vi "rad7_subvi.vi"(8 "error in (no error)":errorcluster, 11 "VISA resource name":refnum<visa-resource-name>) -> (0 "error out":errorcluster, 1 "Rad7 data":dbl, 2 "Rad7 data":string, 3 "VISA resource name out":refnum<visa-resource-name>)   [LabVIEW 2012]
panel:
  out "Numeric 3":i32
  out "read buffer":string
  out "millisecond timer value":u32
  out "Numeric 2":i32
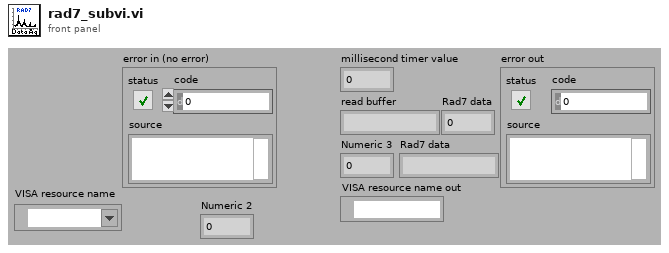
[diagram p1: front panel]
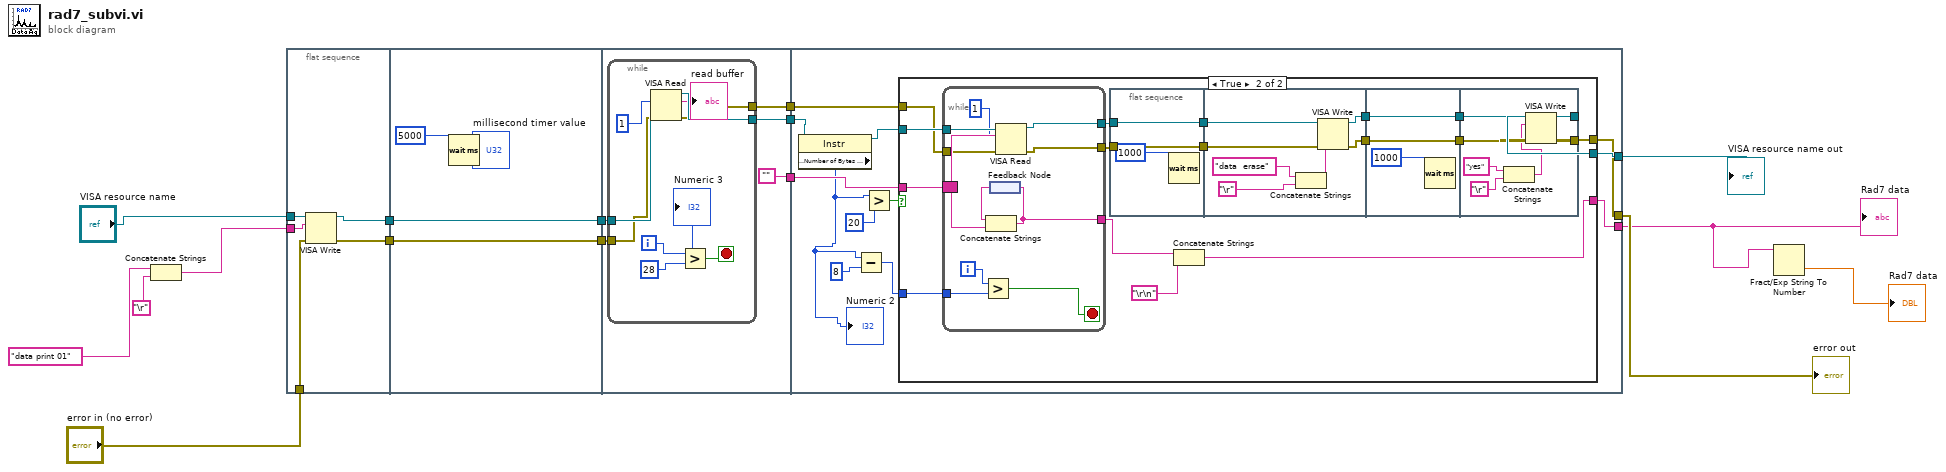
[diagram p0: block diagram]
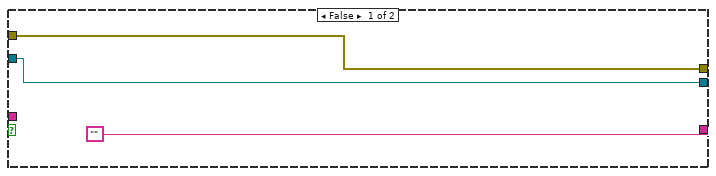
[diagram p2: hidden frame]
diagram:
  n1 = Concatenate Strings("data print 01" ("Command"), "\r") -> (w7:string)
  n2 = flat-sequence {
    tunnel: w7 -> [w21]
    tunnel: [w20] -> w16
    tunnel: [w19] -> w15
    tunnel: "error in (no error)" -> [w18]
    tunnel: "VISA resource name" -> [w17]
    tunnel: w16 -> [w25]
    tunnel: [w25] -> w14
    tunnel: w15 -> [w24]
    tunnel: [w24] -> w13
    tunnel: [w30] -> w12
    tunnel: [""] -> w11
    tunnel: [w28] -> w10
    tunnel: w14 -> [w27]
    tunnel: w13 -> [w26]
    tunnel: [w51] -> w5
    tunnel: w12 -> [w49]
    tunnel: w11 -> [w50]
    tunnel: [w43] -> w2
    tunnel: w10 -> [w45]
    tunnel: [w44] -> w6
    frame #0 {
      n3 = VISA Write(VISA resource name=w17, write buffer=w21, error in (no error)=w18) -> (VISA resource name out=w20:refnum<visa-resource-name>, error out=w19:errorcluster)  [unwired: 1 out]
    }
    frame #1 {
      n4 = Wait (ms)(milliseconds to wait=5000) -> (millisecond timer value=→"millisecond timer value":u32)
    }
    frame #2 {
      n5 = while {
        tunnel: w27 -> [w38]
        tunnel: [w34] -> w30
        tunnel: w26 -> [w33]
        tunnel: [w32] -> w28
        i -> [w37]
        stop <- w35 stop-if-true
        n6 = VISA Read(VISA resource name=w38, byte count=1, error in (no error)=w33) -> (VISA resource name out=w34:refnum<visa-resource-name>, read buffer=→"read buffer":string, error out=w32:errorcluster)  [unwired: 1 out]
        n7 = Greater?(x=w37, y=28) -> (0:w35:bool)
        "Numeric 3" <- w37
      }
    }
    frame #3 {
      n8 = property class="Instr"(reference=w49) -> (reference out=w48:refnum<visa-resource-name>, "Serial Settings:Number of Bytes at Serial Port"=w40:u32)  [unwired: 1 in, 1 out]
      "Numeric 2" <- w40
      n9 = Subtract(x=w40, y=8) -> (x-y=w41:u32)
      n10 = Greater?(x=w40, y=20) -> (0:w47:bool)
      n11 = case shown="True" w47 {
        tunnel: [w54 w65] -> w51
        tunnel: w50 -> [_ w71]
        tunnel: ["" w57] -> w43
        tunnel: w48 -> [w54 w70]
        tunnel: w41 -> [_ w69]
        tunnel: w45 -> [w53 w64]
        tunnel: [w53 w62] -> w44
        frame False {
        }
        frame True {
          n12 = while {
            tunnel: w70 -> [w98]
            border: w71 -> [_]
            tunnel: [w99] -> w67
            tunnel: w69 -> [w96]
            tunnel: [w94] -> w66
            tunnel: w64 -> [w93]
            tunnel: [w92] -> w63
            i -> [w100]
            stop <- w95 stop-if-true
            n13 = Greater?(x=w100, y=w96) -> (0:w95:bool)
            n14 = feedback #1() -> (w101:string)
            n15 = VISA Read(VISA resource name=w98, byte count=1, error in (no error)=w93) -> (VISA resource name out=w94:refnum<visa-resource-name>, read buffer=w102:string, error out=w92:errorcluster)  [unwired: 1 out]
            n16 = Concatenate Strings(w101, w102) -> (w99:string)
            n17 = feedback-in #1(w99) -> ()
          }
          n18 = flat-sequence {
            tunnel: w63 -> [w73]
            tunnel: w66 -> [w74]
            tunnel: [w74] -> w56
            tunnel: [w73] -> w55
            tunnel: [w78] -> w61
            tunnel: [w75] -> w59
            tunnel: w56 -> [w77]
            tunnel: w55 -> [w76]
            tunnel: w61 -> [w84]
            tunnel: [w84] -> w60
            tunnel: w59 -> [w83]
            tunnel: [w83] -> w58
            tunnel: w60 -> [w88]
            tunnel: [w87] -> w65
            tunnel: w58 -> [w86]
            tunnel: [w85] -> w62
            frame #0 {
              n19 = Wait (ms)(milliseconds to wait=1000) -> ()  [unwired: 1 out]
            }
            frame #1 {
              n20 = Concatenate Strings("data  erase", "\r") -> (w79:string)
              n21 = VISA Write(VISA resource name=w77, write buffer=w79, error in (no error)=w76) -> (VISA resource name out=w78:refnum<visa-resource-name>, error out=w75:errorcluster)  [unwired: 1 out]
            }
            frame #2 {
              n22 = Wait (ms)(milliseconds to wait=1000) -> ()  [unwired: 1 out]
            }
            frame #3 {
              n23 = Concatenate Strings("yes", "\r") -> (w89:string)
              n24 = VISA Write(VISA resource name=w88, write buffer=w89, error in (no error)=w86) -> (VISA resource name out=w87:refnum<visa-resource-name>, error out=w85:errorcluster)  [unwired: 1 out]
            }
          }
          n25 = Concatenate Strings(w67, "\r\n") -> (w57:string)
        }
      }
    }
  }
  n26 = Fract/Exp String To Number(string=w2) -> (number=→"Rad7 data":dbl)  [unwired: 3 in, 1 out]
  "Rad7 data" <- w2
  "VISA resource name out" <- w5
  "error out" <- w6
